vi "Data_Base_logging.vi"(0 "Rig Setup":string) -> (1 "Logging On?":bool, 2 "Close Loop with Pitot?":bool, 3 "Rig Name":string, 4 "DB Setup files":string[](array[string])=["EnFlo_Tunnel DB setup.xls", "A_Tunnel DB setup.xls", "D_Tunnel DB setup.xls", "Aero_Tunnel DB setup.xls", "CPP_GDE DB setup.xls", "CPP_GDW DB setup.xls", "CPP_GDRT DB setup.xls"] caption="DB Setup files (from EnFlo Tun Setup Global)")   [LabVIEW 2022 SP3]
uses:
  Controls/Server_Comms.ctl
  Globals/Preference_global.vi
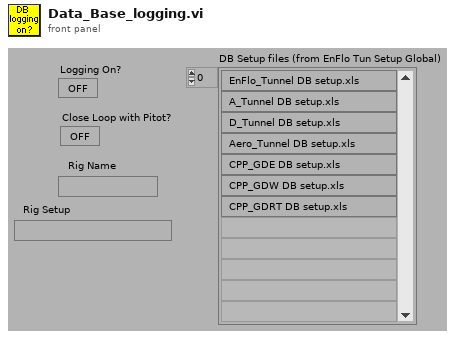
[diagram p1: front panel]
types:
  T1 = typedef "Server_Comms.ctl" = enum16{"Do Not Link To Server", "Server Link Healthy"}
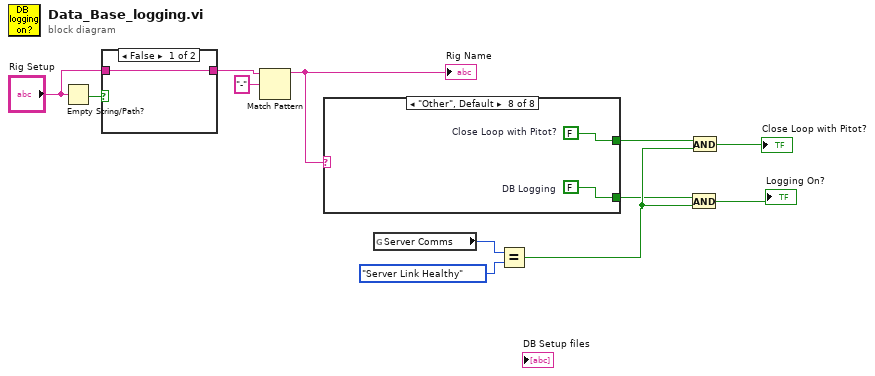
[diagram p0: block diagram]
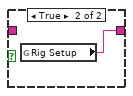
[diagram p2: hidden frame]
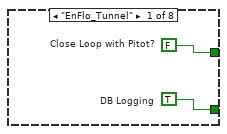
[diagram p3: hidden frame]
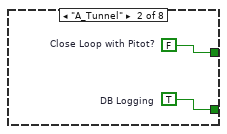
[diagram p4: hidden frame]
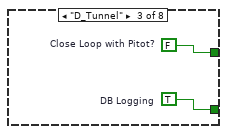
[diagram p5: hidden frame]
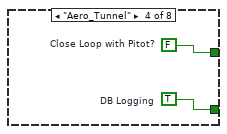
[diagram p6: hidden frame]
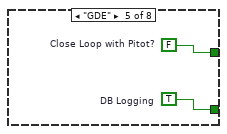
[diagram p7: hidden frame]
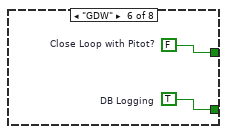
[diagram p8: hidden frame]
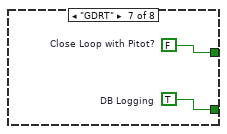
[diagram p9: hidden frame]
diagram:
  n1 = Empty String/Path?(string/path="Rig Setup") -> (empty?=w3:bool)
  n2 = case shown="False" w3 {
    tunnel: [w13 w14] -> w2
    tunnel: "Rig Setup" -> [w13 _]
    frame False {
    }
    frame True {
      n3 = global read "Preference_global.vi" "Rig Setup"() -> (w14:string)
    }
  }
  n4 = Match Pattern(string=w2, regular expression="-") -> (before substring=w4:string)  [unwired: 4 out]
  "Rig Name" <- w4
  n5 = case shown="\"Other\", Default" w4 {
    tunnel: [w16 w18 w20 w22 w24 w26 w28 w30] -> w7
    tunnel: [w15 w17 w19 w21 w23 w25 w27 w29] -> w6
    frame "EnFlo_Tunnel" {
      w15 = TRUE  # DB Logging
      w16 = FALSE  # Close Loop with Pitot?
    }
    frame "A_Tunnel" {
      w17 = TRUE  # DB Logging
      w18 = FALSE  # Close Loop with Pitot?
    }
    frame "D_Tunnel" {
      w19 = TRUE  # DB Logging
      w20 = FALSE  # Close Loop with Pitot?
    }
    frame "Aero_Tunnel" {
      w21 = TRUE  # DB Logging
      w22 = FALSE  # Close Loop with Pitot?
    }
    frame "GDE" {
      w23 = TRUE  # DB Logging
      w24 = FALSE  # Close Loop with Pitot?
    }
    frame "GDW" {
      w25 = TRUE  # DB Logging
      w26 = FALSE  # Close Loop with Pitot?
    }
    frame "GDRT" {
      w27 = TRUE  # DB Logging
      w28 = FALSE  # Close Loop with Pitot?
    }
    frame "Other", Default {
      w29 = FALSE  # DB Logging
      w30 = FALSE  # Close Loop with Pitot?
    }
  }
  n6 = global read "Preference_global.vi" "Server Comms"() -> (w11:T1)
  n7 = Equal?(x=w11, y=Server_Comms."Server Link Healthy" ("Server Comms")) -> (x = y?=w8:bool)
  n8 = And(x=w6, y=w8) -> (x .and. y?=→"Logging On?":bool)
  n9 = And(x=w7, y=w8) -> (x .and. y?=→"Close Loop with Pitot?":bool)
